vi "Count_Events.vi"(8 "error in (no error)":errorcluster, 10 "Small?":bool, 11 "Constraints":T1 {"Estimate Quality" scale=0.0..5.0; "Lower Mass Limit (kg)" min=-1.0 max=1.0 step=1e-20; "Upper Mass Limit (kg)" min=-1.0 max=1.0 step=1e-20; "Lower Velocity Limit (km/s)" min=-1.0 max=299792000.0; "Upper Velocity Limit (km/s)" min=-1.0 max=299792000.0}) -> (0 "error out":errorcluster, 3 "Number of Events":i64)   [LabVIEW 2013]
uses:
  Controls/Constraints.ctl
  <vilib>/addons/database/Auxilliary.llb/DB Tools Cursor Type.ctl
  <userlib>/_OpenG.lib/array/array.llb/Remove Duplicates from 1D Array (String)__ogtk.vi
  <userlib>/_OpenG.lib/array/array.llb/Search 1D Array (String)__ogtk.vi
  <userlib>/_OpenG.lib/array/array.llb/Delete Elements from 1D Array (String)__ogtk.vi
  <vilib>/addons/database/Connection.llb/Conn Execute.vi
  <vilib>/addons/database/Recordset.llb/Rec Fetch Recordset Data (R).vi
  <userlib>/_OpenG.lib/array/array.llb/Empty 2D Array (Variant)__ogtk.vi
  <vilib>/addons/database/Recordset.llb/Rec Destroy - Connection.vi
  <vilib>/addons/database/_DB Variant To Data/Database Variant To Data.xnode
  <vilib>/addons/database/NI_Database_API.lvlib
panel:
  out "Count Events Syntax":string
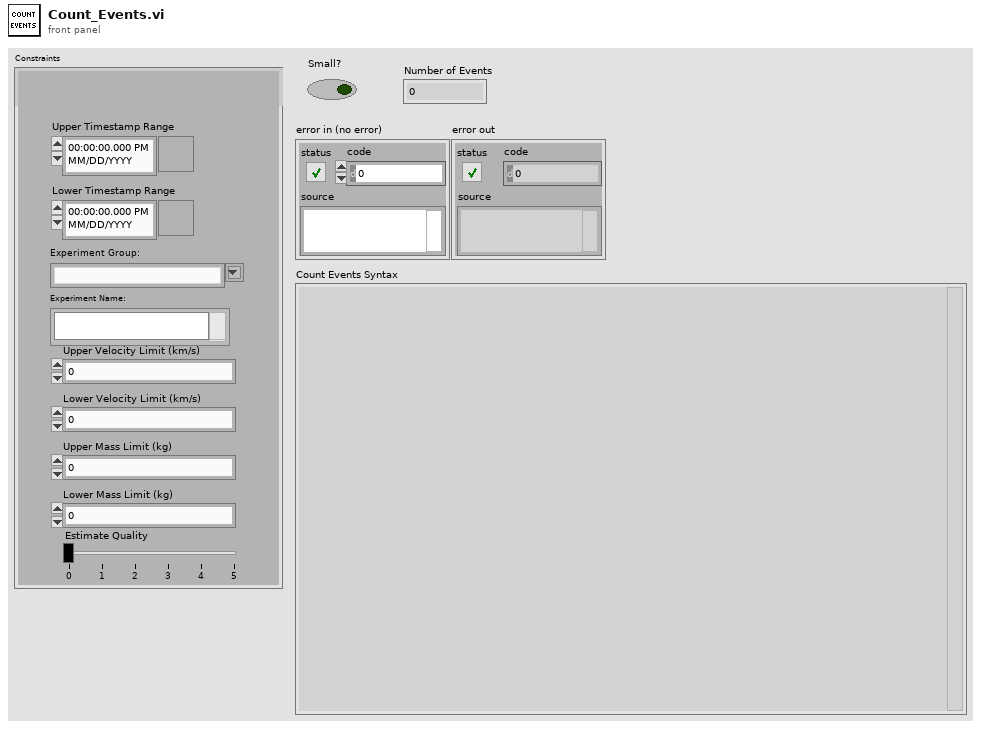
[diagram p1: front panel]
types:
  T1 = typedef "Constraints.ctl" = cluster{"Upper Timestamp Range":timestamp, "Lower Timestamp Range":timestamp, "Experiment Group:":string, "Experiment Name:":i32[], "Upper Velocity Limit (km/s)":dbl, "Lower Velocity Limit (km/s)":dbl, "Upper Mass Limit (kg)":dbl, "Lower Mass Limit (kg)":dbl, "name array":string[], "Estimate Quality":cluster{dbl, dbl}}
  T2 = typedef "NI_Database_API.lvlib/DB Tools Cursor Type.ctl" = enum16{"forward-only", "keyset", "dynamic", "static"}
  T3 = typedef "NI_Database_API.lvlib/Conn ObjectReference.ctl" = refnum<k1>
  T4 = typedef "NI_Database_API.lvlib/Rec ObjectReference.ctl" = refnum<k1>
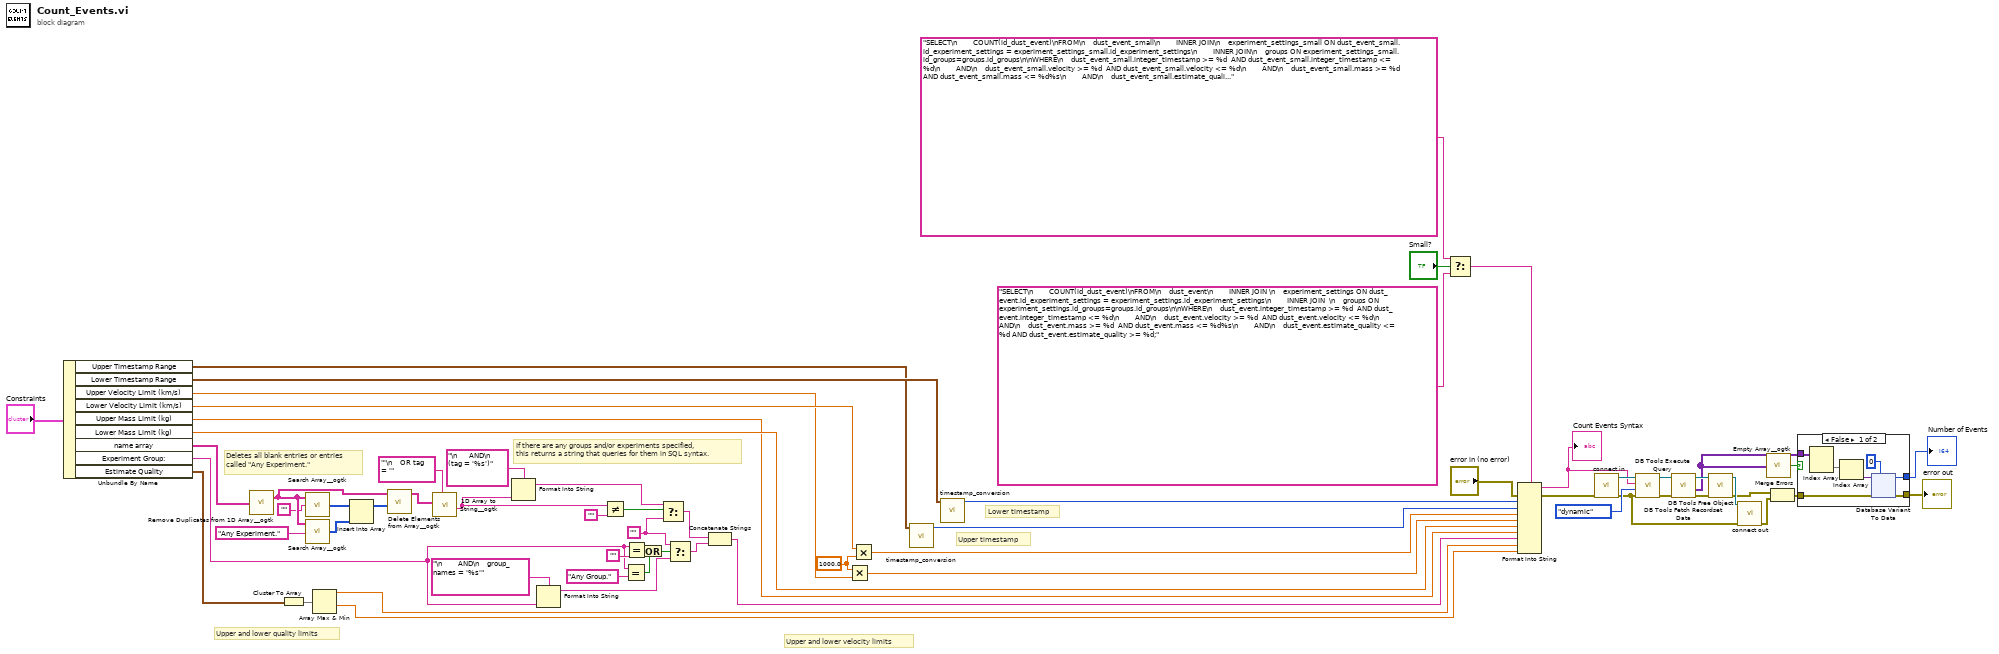
[diagram p0: block diagram]
diagram:
  w31 = 1000.0 ("y")
  w64 = ""
  # "Upper and lower velocity limits"
  # "Deletes all blank entries or entries\ncalled \"Any Experiment.\""
  # "Upper and lower quality limits"
  # "Upper timestamp"
  # "Lower timestamp"
  # "If there are any groups and/or experiments specified,\nthis returns a string that queries for them in SQL syntax."
  n1 = Unbundle By Name("Constraints") -> ("Upper Timestamp Range"=w9:timestamp, "Lower Timestamp Range"=w10:timestamp, "Upper Velocity Limit (km/s)"=w11:dbl, "Lower Velocity Limit (km/s)"=w12:dbl, "Upper Mass Limit (kg)"=w13:dbl, "Lower Mass Limit (kg)"=w14:dbl, "name array"=w16:string[], "Experiment Group:"=w15:string, "Estimate Quality"=w24:cluster{dbl, dbl})
  n2 = call-poly <userlib>:"Remove Duplicates from 1D Array__ogtk.vi"("Input Array"=w16) -> ("Output Array"=w59:string[])  [unwired: 1 out]
  n3 = Cluster To Array(cluster=w24) -> (array=w32:dbl[])
  n4 = call-poly <userlib>:"Search Array__ogtk.vi"("Array"=w59, "Element Data"="") -> ("Indices of Elements"=w36:i32[])  [unwired: 7 in]
  n5 = call-poly <userlib>:"Search Array__ogtk.vi"("Array"=w59, "Element Data"="Any Experiment.") -> ("Indices of Elements"=w61:i32[])  [unwired: 7 in]
  n6 = Array Max & Min(array=w32) -> (max value=w57:dbl, min value=w56:dbl)  [unwired: 2 out]
  n7 = Insert Into Array(array=w36, new element=w61) -> (w60:i32[])  [unwired: 1 in]
  n8 = call-poly <userlib>:"Delete Elements from Array__ogtk.vi"("indices"=w60, "array"=w59) -> ("array w/ subset deleted"=w37:string[])  [unwired: 8 in, 1 out]
  n9 = call <userlib>:"1D Array to String__ogtk.vi"("delimiter (Tab)"="'\n    OR tag = '", "Array of Strings"=w37) -> ("delimited string"=w43:string)  [unwired: 9 in]
  n10 = Format Into String(format string="\n      AND\n    (tag = '%s')" ("string"), w43) -> (resulting string=w63:string)  [unwired: 2 in, 1 out]
  n11 = Format Into String(format string="\n        AND\n    group_names = '%s'" ("string"), w15) -> (resulting string=w29:string)  [unwired: 2 in, 1 out]
  n12 = Not Equal?(x=w43, y="") -> (x != y?=w62:bool)
  n13 = Equal?(x=w15, y="Any Group.") -> (x = y?=w38:bool)
  n14 = Equal?(x=w15, y="") -> (x = y?=w41:bool)
  n15 = Or(x=w41, y=w38) -> (x .or. y?=w40:bool)
  n16 = Select(t=w63, s=w62, f=w64) -> (s? t:f=w26:string)
  n17 = Select(t=w64, s=w40, f=w29) -> (s? t:f=w27:string)
  n18 = Concatenate Strings(w26, w27) -> (w55:string)
  n19 = Multiply(x=w31, y=w11) -> (x*y=w54:dbl)
  n20 = Multiply(x=w12, y=w31) -> (x*y=w53:dbl)
  n21 = call "timestamp_conversion.vi"("Time Stamp"=w9) -> ("Integer Time"=w52:i64)  [unwired: 8 in, 1 out]
  n22 = call "timestamp_conversion.vi"("Time Stamp"=w10) -> ("Integer Time"=w51:i64)  [unwired: 8 in, 1 out]
  n23 = Select(t="SELECT\n        COUNT(id_dust_event)\nFROM\n    dust_event_small\n        INNER JOIN\n    experiment_settings_small ON dust_event_small.id_experiment_settings = experiment_settings_small.id_experiment_settings\n        INNER JOIN\n    groups ON experiment_settings_small.id_groups=groups.id_groups\n\nWHERE\n    dust_event_small.integer_timestamp >= %d  AND dust_event_small.integer_timestamp <= %d\n        AND\n    dust_event_small.velocity >= %d  AND dust_event_small.velocity <= %d\n        AND\n    dust_event_small.mass >= %d  AND dust_event_small.mass <= %d%s\n        AND\n    dust_event_small.estimate_quality <= %d AND dust_event_small.estimate_quality >= %d;" ("string"), s="Small?", f="SELECT\n        COUNT(id_dust_event)\nFROM\n    dust_event\n        INNER JOIN \n    experiment_settings ON dust_event.id_experiment_settings = experiment_settings.id_experiment_settings\n        INNER JOIN  \n    groups ON experiment_settings.id_groups=groups.id_groups\n\nWHERE\n    dust_event.integer_timestamp >= %d  AND dust_event.integer_timestamp <= %d\n        AND\n    dust_event.velocity >= %d  AND dust_event.velocity <= %d\n        AND\n    dust_event.mass >= %d  AND dust_event.mass <= %d%s\n        AND\n    dust_event.estimate_quality <= %d AND dust_event.estimate_quality >= %d;" ("string")) -> (s? t:f=w2:string)
  n24 = Format Into String(format string=w2, error in="error in (no error)", w51, w52, w53, w54, w14, w13, w55, w57, w56) -> (resulting string=w1:string, error out=w46:errorcluster)  [unwired: 1 in]
  "Count Events Syntax" <- w1
  n25 = call "connect in.vi"("error in (no error)"=w46) -> ("error out"=w17:errorcluster, "Database Connection"=w47:T3)  [unwired: 6 in, 1 out]
  n26 = call-poly <vilib>:"DB Tools Execute Query.vi"("error in (no error)"=w17, "cursor type"=DB_Tools_Cursor_Type."dynamic", "SQL query"=w1, "connection reference"=w47) -> ("error out"=w50:errorcluster, "recordset reference"=w49:T4)  [unwired: 4 in]
  n27 = call-poly <vilib>:"DB Tools Fetch Recordset Data.vi"("error in (no error)"=w50, "recordset reference"=w49) -> ("error out"=w45:errorcluster, "recordset data"=w23:variant[][], "recordset reference out"=w48:T4)  [unwired: 3 in]
  n28 = call-poly <vilib>:"DB Tools Free Object.vi"("error in (no error)"=w45, "recordset reference"=w48) -> ("error out"=w21:errorcluster, "connection reference"=w22:T3)  [unwired: 8 in]
  n29 = call "connect out.vi"("error in (no error)"=w17, "connection reference"=w22) -> ("error out"=w20:errorcluster)  [unwired: 9 in]
  n30 = call-poly <userlib>:"Empty Array__ogtk.vi"("Array"=w23) -> ("Empty Array?"=w18:bool)  [unwired: 8 in]
  n31 = Merge Errors(w21, w20) -> (w19:errorcluster)
  n32 = case shown="False" w18 {
    tunnel: w23 -> [w71 _]
    tunnel: w19 -> [w68 w104]
    tunnel: [w67 w104] -> w7
    tunnel: [w66 _] -> w6
    frame False {
      n33 = Index Array(array=w71) -> (element=w70:variant[])  [unwired: 2 in]
      n34 = Index Array(array=w70) -> (element=w69:variant)  [unwired: 1 in]
      n35 = xnode "Database Variant To Data"("database variant"=w69, "error in (no error)"=w68, "type"=i64 0 ("Number of Events")) -> ("data"=w66:i64, "error out"=w67:errorcluster)
    }
    frame True {
    }
  }
  "error out" <- w7
  "Number of Events" <- w6
